vi "OAT Spectral Map (Waterfall).vi"(0 "scaled signal [EU]":waveform(dbl)={"t0"=timestamp(0 s since 1904-01-01), "dt"=0.0, "Y"=[]}, 1 "dB on? (F)":bool, 2 "reset? (F)":bool, 3 "plot type":T10(ring), 5 "speed profile":T9 {"speed [RPM]" format="%.2f"; "time [s]" format="%.2f"}, 7 "pulse/revolution (1)":i32=1, 9 "time/speed segment [s or RPM]":cluster{"start":dbl, "end":dbl, "step size":dbl} {"step size" format="%.2f"; "end" min=0.0 format="%.2f"; "start" min=0.0 format="%.2f"}, 11 "error in (no error)":errorcluster, 12 "max order (auto)":dbl, 13 "windows info":cluster{"window type":u32, "window length":i32}={"window type"=62, "window length"=2048} {"window length" min=2; "window type" items=["None"=0, "Hanning"=1, "Hamming"=2, "Blackman-Harris"=3, "Exact Blackman"=4, "Blackman"=5, "Flat Top"=6, "4 Term B-Harris"=7, "7 Term B-Harris"=8, "Low Sidelobe"=9, "Gaussian"=62]}) -> (4 "waterfall graph":T1, 6 "waterfall unit labels":T8, 8 "spectrum info":T2={"channel name"="", "description"="", "x-axis units"=0, "spectral info"={"spectrum type"=enum."Power [Magnitude^2]", "linear/dB"=enum."linear", "window"=0, "window size"=0, "FFT size"=0}, "engineering units"=0, "custom label"="", "dB reference [EU]"=0.0, "peak units"=enum."rms", "weighting filter"=0, "spectral density?"=FALSE, "unit label"="", "spectrum skewed?"=FALSE, "complimentary spectrum units"=enum."none"} {"x-axis units" items=["Time (s)"=0, "Frequency-CB (Hz)"=1, "Frequency-CPB (Hz)"=1248, "Frequency-Arbitrary (Hz)"=2357, "Quefrency (s)"=2, "Revolutions (rev)"=3, "Order"=4, "Speed (RPM)"=11, "Speed (rad/s)"=21, "Index"=65535]; "weighting filter" items=["Linear", "A-weighting", "B-weighting", "C-weighting", "ITU-R 468-4", "Dolby", "CCITT", "C-message", "Wb", "Wc", "Wd", "We", "Wf", "Wh", "Wj", "Wk", "Wm", "AES17 20 kHz lowpass", "AES17 40 kHz lowpass", "AES17 20 kHz highpass", "AES17 40 kHz highpass"]; "dB reference [EU]" format="%.2f"; "engineering units" items=["custom..."=0, "V"=1, "A"=21, "C"=30, "pC"=31, "s"=32, "-"=29, "Pa"=2, "N"=20, "g"=3, "m/s^2"=4, "m/s"=5, "m"=6, "mm/s"=12, "mm"=13, "micron/s"=14, "micron"=15, "in/s^2"=7, "in/s"=8, "in"=9, "mil/s"=10, "mil"=11, "rad/s^2"=16, "rad/s"=17, "rad"=18, "deg/s^2"=26, "deg/s"=27, "deg"=28, "RPM"=22, "cycle/s^2"=23, "Hz"=24, "cycle"=25, "strain"=19]; "spectral info"."window" items=["None "=0, "Hanning"=1, "Hamming"=2, "Blackman-Harris"=3, "Exact Blackman"=4, "Blackman"=5, "Flat Top"=6, "4 Term B-Harris "=7, "7 Term B-Harris"=8, "Low Sidelobe"=9, "Force - Exponential"=10, "Gaussian"=62]}, 10 "end reached?":bool, 15 "error out":errorcluster)   [LabVIEW 2017, in "SoundVib_OrderTracking.lvlib"]
doc: "Computes a spectral map of the <B>scaled signal [EU]</B> as a function of time or rotational speed. This VI can return the spectral map as a 2D numeric array, a colormap, or a waterfall graph. Wire data to the <B>scaled signal [EU]</B> input to determine the polymorphic instance to use or manually select the instance."
uses:
  <vilib>/addons/Sound and Vibration/Order Analysis/Resample Order Tracking/SoundVib_OrderTracking.lvlib
  <vilib>/addons/Sound and Vibration/Order Analysis/Tach Process/SubVIs/speed profile.ctl
  <vilib>/addons/_NISVFA/_Shared subVIs/Controls/svc_Spectrum Info.ctl
  <vilib>/addons/_NISVFA/_Shared subVIs/Controls/svc_X-Axis Units.ctl
  <vilib>/addons/_NISVFA/_Shared subVIs/Controls/svc_Spectrum Type.ctl
  <vilib>/addons/_NISVFA/_Shared subVIs/Controls/svc_Engineering Units Text Ring.ctl
  <vilib>/addons/_NISVFA/_Shared subVIs/Controls/svc_Weighting Filter Text Ring.ctl
  <vilib>/addons/_NISVFA/_Shared subVIs/Controls/svc_Complimentary Spectrum Units.ctl
  <vilib>/addons/_NISVFA/_Shared subVIs/Common/svc_Check for Waveform Parameter Continuity (no state).vi
  <vilib>/addons/Sound and Vibration/Order Analysis/Resample Order Tracking/OAT Convert to Even Angle Signal (1 Channel).vi
  <vilib>/Waveform/WDTOps.llb/WDT Waveform Duration DBL.vi
  <vilib>/addons/_NISVFA/_Shared subVIs/Common/svc_Engineering Units to Unit Label.vi
  <vilib>/addons/_NISVFA/_Shared subVIs/Common/svc_Unit Label to Engineering Units.vi
  <vilib>/addons/Sound and Vibration/Order Analysis/Resample Order Tracking/SoundVib_Resampling.lvlib
  <vilib>/addons/Sound and Vibration/Order Analysis/Tach Process/SoundVib_TachProcess.lvlib
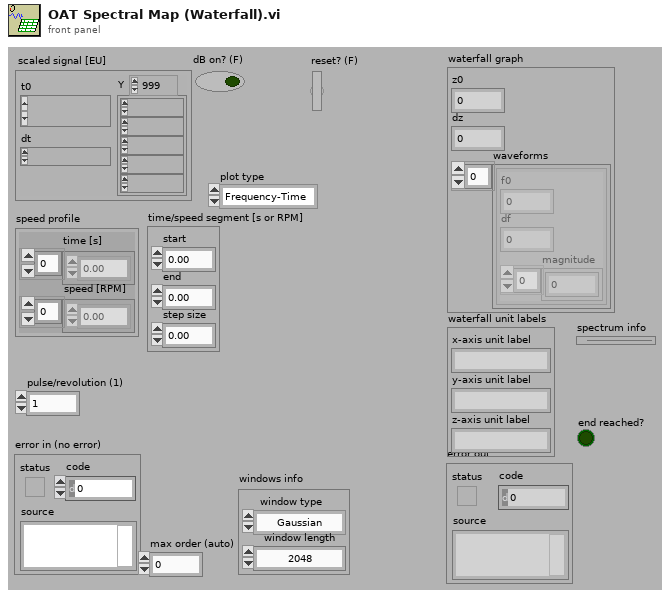
[diagram p1: front panel]
types:
  T1 = cluster{"z0":dbl, "dz":dbl, "waveforms":cluster{"f0":dbl, "df":dbl, "magnitude":dbl[]}[]}
  T2 = typedef "svc_Spectrum Info.ctl" = cluster{"channel name":string, "description":string, "x-axis units":T3, "spectral info":cluster{"spectrum type":T4, "linear/dB":enum16{"linear", "dB"}, "window":u16, "window size":i32, "FFT size":i32}, "engineering units":T5, "custom label":string, "dB reference [EU]":dbl, "peak units":enum16{"rms", "peak", "peak-peak"}, "weighting filter":T6, "spectral density?":bool, "unit label":string, "spectrum skewed?":bool, "complimentary spectrum units":T7}
  T3 = typedef "svc_X-Axis Units.ctl" = u16
  T4 = typedef "svc_Spectrum Type.ctl" = enum16{"FFT Spectrum [complex]", "Amplitude [Magnitude]", "Power [Magnitude^2]", "Cross Spectrum [complex]", "Frequency Response [Complex]"}
  T5 = typedef "svc_Engineering Units Text Ring.ctl" = u16
  T6 = typedef "svc_Weighting Filter Text Ring.ctl" = u16
  T7 = typedef "svc_Complimentary Spectrum Units.ctl" = enum16{"none", "radians", "degrees", "cycles", "imaginary"}
  T8 = cluster{"x-axis unit label":string, "y-axis unit label":string, "z-axis unit label":string}
  T9 = typedef "SoundVib_TachProcess.lvlib/speed profile.ctl" = cluster{"time [s]":dbl[], "speed [RPM]":dbl[]}
  T10 = enum16{"Frequency-Time", "Time-Frequency", "Order-Time", "Time-Order", "Frequency-RPM", "RPM-Frequency", "Order-RPM", "RPM-Order"}
  T11 = cluster{"dt":bool, "t0 continuity":bool, "array length":bool, "channel info":bool, "name":bool}
  T12 = cluster{"start (s)":dbl, "end (s)":dbl, "step (s)":dbl}
  T13 = typedef "svc_Channel Info.ctl" = cluster{"sensor sensitivity":dbl, "engineering units":T5, "dB reference":dbl, "custom label":string, "weighting filter":T6, "pregain":dbl}
  T14 = cluster{"X scale":cluster{"offset":dbl, "multiplier":dbl}, "Y scale":cluster{"offset":dbl, "multiplier":dbl}}
  T15 = cluster{"X axis unit label":string, "Y axis unit label":string, "Z axis unit label":string}
  T16 = cluster{"z0":dbl, "dz":dbl, "Waveforms":cluster{"f0":dbl, "df":dbl, "magnitude":dbl[]}[]}
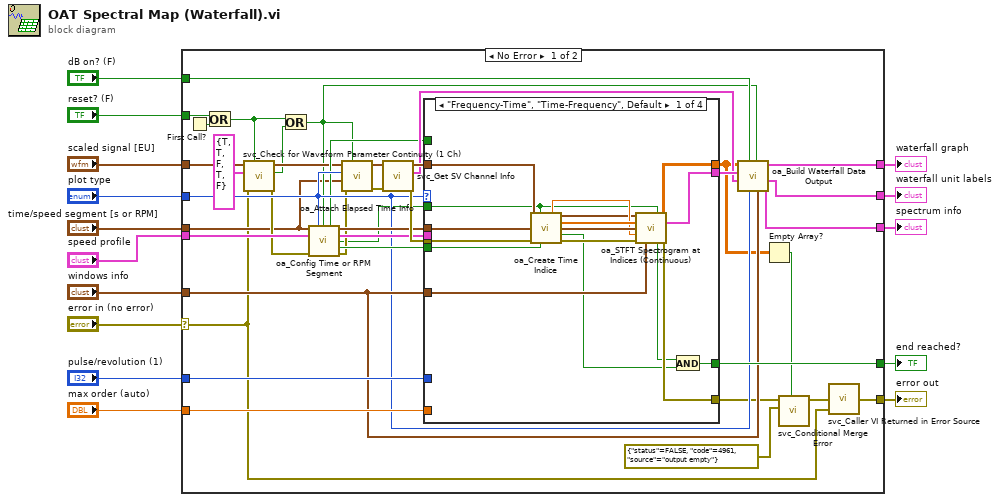
[diagram p0: block diagram]
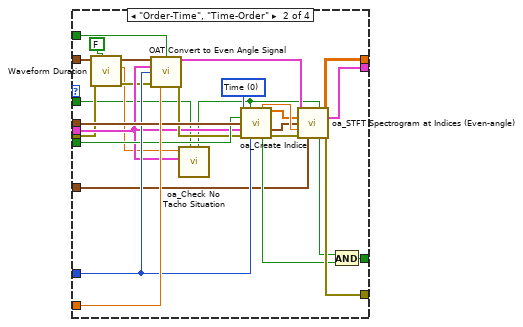
[diagram p2: hidden frame]
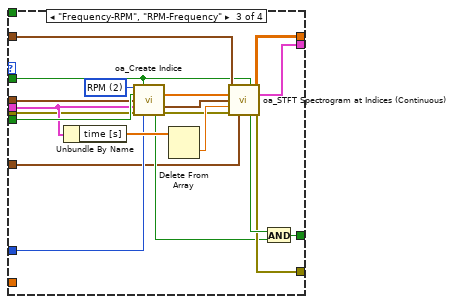
[diagram p3: hidden frame]
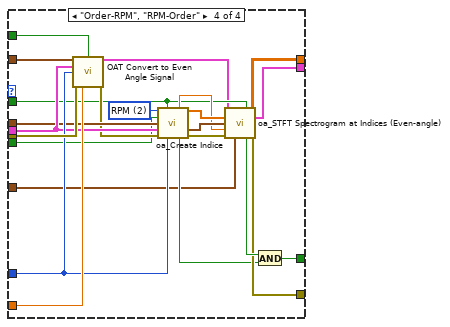
[diagram p4: hidden frame]
diagram:
  n1 = case shown="No Error" "error in (no error)" {
    selector: "error in (no error)" -> [w18 w143]
    tunnel: [w16 w143] -> w15
    tunnel: "time/speed segment [s or RPM]" -> [w23 _]
    tunnel: "scaled signal [EU]" -> [w30 _]
    tunnel: [w54 _] -> w12
    tunnel: "windows info" -> [w37 _]
    tunnel: "speed profile" -> [w41 _]
    tunnel: "pulse/revolution (1)" -> [w53 _]
    tunnel: "max order (auto)" -> [w52 _]
    tunnel: "reset? (F)" -> [w51 _]
    tunnel: "dB on? (F)" -> [w50 _]
    tunnel: [w49 _] -> w1
    tunnel: "plot type" -> [w35 _]
    tunnel: [w47 _] -> w3
    tunnel: [w46 _] -> w2
    frame No Error {
      n2 = First Call?() -> (First Call?: T/F=w48:bool)
      n3 = Or(x=w51, y=w48) -> (x .or. y?=w26:bool)
      n4 = call <vilib>:"svc_Check for Waveform Parameter Continuity (1 Ch).vi"("restart averaging (F)"=w26, "error in (no error)"=w18, "checks for channel parameter change"=T11 {"dt"=TRUE, "t0 continuity"=TRUE, "array length"=FALSE, "channel info"=TRUE, "name"=FALSE}, "scaled signal [EU]"=w30) -> ("error out"=w29:errorcluster, "waveform parameter changed"=w25:bool, "dup scaled signal [EU]"=w28:waveform(dbl))  [unwired: 2 in, 3 out]
      n5 = Or(x=w26, y=w25) -> (x .or. y?=w24:bool)
      n6 = call <vilib>:"oa_Config Time or RPM Segment.vi"("time segment"=w23, "plot type"=w35, "reset in"=w24, "speed profile"=w41, "error in (no error)"=w29) -> ("reset resampling"=w31:bool, "time segment out"=w40:T12, "speed profile out"=w39:T9, "reset out"=w32:bool, "step found?"=w38:bool, "error out"=w34:errorcluster)  [unwired: 5 in]
      n7 = call <vilib>:"oa_Attach Elapsed Time Info.vi"("reset? (F)"=w24, "error in (no error)"=w34, "time/speed segment [s or rpm]"=w23, "plot type"=w35, "scaled signal [EU]"=w28) -> ("error out"=w33:errorcluster, "scaled signal [EU] out"=w36:waveform(dbl))  [unwired: 5 in]
      n8 = call <vilib>:"svc_Get SV Channel Info.vi"("error in (no error)"=w33, "scaled signal [EU]"=w36) -> ("error out"=w44:errorcluster, "channel info"=w42:T13, "dup scaled signal [EU]"=w45:waveform(dbl))  [unwired: 4 in, 3 out]
      n9 = case shown="\"Frequency-Time\", \"Time-Frequency\", Default" w35 {
        tunnel: w45 -> [w57 w95 w106 w135]
        tunnel: w40 -> [w63 w88 w112 w130]
        tunnel: [w71 w97 w118 w142] -> w20
        tunnel: [w70 w96 w117 w141] -> w43
        tunnel: [w69 w98 w115 w138] -> w21
        tunnel: [w67 w93 w116 w139] -> w54
        tunnel: w44 -> [w56 w77 w102 w137]
        tunnel: w39 -> [_ w79 w111 w131]
        tunnel: w53 -> [_ w87 w105 w132]
        tunnel: w52 -> [_ w99 _ w136]
        tunnel: w38 -> [w64 w86 w114 w124]
        tunnel: w37 -> [w66 w83 w103 w123]
        tunnel: w32 -> [w55 w73 w100 w122]
        tunnel: w31 -> [_ w81 _ w121]
        frame "Frequency-Time", "Time-Frequency", Default {
          n10 = call <vilib>:"oa_Create Time Indice.vi"("scaled signal [EU]"=w57, "reset? (True)"=w55, "steps"=w63, "error in (no error)"=w56, "step found?(F)"=w64) -> ("signal processed"=w59:dbl, "scaled signal [EU] dup"=w58:waveform(dbl), "time indices"=w62:dbl[], "scale"=w61:cluster{"offset":dbl, "multiplier":dbl}, "finished?"=w60:bool, "error out"=w65:errorcluster)  [unwired: 5 in]
          n11 = call <vilib>:"oa_STFT Spectrogram at Indices (Continuous).vi"("resampled signal"=w58, "reset? (True)"=w55, "time indices"=w62, "X scale in"=w61, "last indices"=w59, "error in (no error)"=w65, "spectral settings"=w66) -> ("spectral map"=w71:dbl[][], "scales"=w70:T14, "finished"=w68:bool, "error out"=w69:errorcluster)  [unwired: 5 in]
          n12 = And(x=w68, y=w60) -> (x .and. y?=w67:bool)
        }
        frame "Order-Time", "Time-Order" {
          w92 = u16 0 items=["Time", "Revolution", "RPM"] ("X axis selection")
          n13 = call-poly <vilib>:"Waveform Duration.vi"("open interval? (T)"=FALSE, "error in (no error)"=w77, "waveform in"=w95) -> ("error out"=w76:errorcluster, "duration"=w74:dbl, "waveform out"=w78:waveform(dbl))  [unwired: 6 in]
          n14 = call-poly <vilib>:"OAT Convert to Even Angle Signal.vi"("scaled signal [EU]"=w78, "reset? (F)"=w81, "speed profile"=w79, "pulse/revolution (1)"=w87, "error in (no error)"=w76, "max order (auto)"=w99) -> ("even-angle signal"=w80:cluster{"r0":dbl, "dr":dbl, "Y":dbl[]}, "error out"=w85:errorcluster)  [unwired: 5 in, 3 out]
          n15 = call <vilib>:"oa_Check No Tacho Situation.vi"("reset in"=w73, "speed profile"=w79, "input duration"=w74) -> ("reset out"=w72:bool)  [unwired: 8 in]
          n16 = call <vilib>:"oa_Create Indice.vi"("X axis selection"=w92, "reset?(F)"=w72, "step found?(F)"=w86, "steps input"=w88, "speed profile"=w79, "error in (no error)"=w85, "pulse/revolution (1)"=w87) -> ("last rev"=w90:dbl, "rev indice"=w82:dbl[], "scale"=w89:cluster{"offset":dbl, "multiplier":dbl}, "reach end?"=w91:bool, "error out"=w84:errorcluster)  [unwired: 2 in, 2 out]
          n17 = call <vilib>:"oa_STFT Spectrogram at Indices (Even-angle).vi"("even-angle signal"=w80, "reset? (True)"=w72, "rev indices"=w82, "X scale in"=w89, "last indices"=w90, "error in (no error)"=w84, "spectral settings"=w83) -> ("spectral map"=w97:dbl[][], "scales"=w96:T14, "finished"=w94:bool, "error out"=w98:errorcluster)  [unwired: 5 in]
          n18 = And(x=w94, y=w91) -> (x .and. y?=w93:bool)
        }
        frame "Frequency-RPM", "RPM-Frequency" {
          w113 = u16 2 items=["Time", "Revolution", "RPM"] ("X axis selection")
          n19 = Unbundle By Name(w111) -> ("time [s]"=w108:dbl[])
          n20 = call <vilib>:"oa_Create Indice.vi"("X axis selection"=w113, "reset?(F)"=w100, "step found?(F)"=w114, "steps input"=w112, "speed profile"=w111, "error in (no error)"=w102, "pulse/revolution (1)"=w105) -> ("time indice"=w110:dbl[], "scale"=w109:cluster{"offset":dbl, "multiplier":dbl}, "reach end?"=w104:bool, "error out"=w101:errorcluster)  [unwired: 2 in, 3 out]
          n21 = Delete From Array(array=w108) -> (deleted portion=w107:dbl)  [unwired: 2 in, 1 out]
          n22 = call <vilib>:"oa_STFT Spectrogram at Indices (Continuous).vi"("resampled signal"=w106, "reset? (True)"=w100, "time indices"=w110, "X scale in"=w109, "last indices"=w107, "error in (no error)"=w101, "spectral settings"=w103) -> ("spectral map"=w118:dbl[][], "scales"=w117:T14, "finished"=w119:bool, "error out"=w115:errorcluster)  [unwired: 5 in]
          n23 = And(x=w119, y=w104) -> (x .and. y?=w116:bool)
        }
        frame "Order-RPM", "RPM-Order" {
          w134 = u16 2 items=["Time", "Revolution", "RPM"] ("X axis selection")
          n24 = call-poly <vilib>:"OAT Convert to Even Angle Signal.vi"("scaled signal [EU]"=w135, "reset? (F)"=w121, "speed profile"=w131, "pulse/revolution (1)"=w132, "error in (no error)"=w137, "max order (auto)"=w136) -> ("even-angle signal"=w120:cluster{"r0":dbl, "dr":dbl, "Y":dbl[]}, "error out"=w126:errorcluster)  [unwired: 5 in, 3 out]
          n25 = call <vilib>:"oa_Create Indice.vi"("X axis selection"=w134, "reset?(F)"=w122, "step found?(F)"=w124, "steps input"=w130, "speed profile"=w131, "error in (no error)"=w126, "pulse/revolution (1)"=w132) -> ("last rev"=w127:dbl, "rev indice"=w128:dbl[], "scale"=w129:cluster{"offset":dbl, "multiplier":dbl}, "reach end?"=w133:bool, "error out"=w125:errorcluster)  [unwired: 2 in, 2 out]
          n26 = call <vilib>:"oa_STFT Spectrogram at Indices (Even-angle).vi"("even-angle signal"=w120, "reset? (True)"=w122, "rev indices"=w128, "X scale in"=w129, "last indices"=w127, "error in (no error)"=w125, "spectral settings"=w123) -> ("spectral map"=w142:dbl[][], "scales"=w141:T14, "finished"=w140:bool, "error out"=w138:errorcluster)  [unwired: 5 in]
          n27 = And(x=w140, y=w133) -> (x .and. y?=w139:bool)
        }
      }
      n28 = call <vilib>:"oa_Build Waterfall Data Output.vi"("windows info"=w37, "reset? (F)"=w24, "plot type"=w35, "dB on"=w50, "channel info"=w42, "scales"=w43, "spectral map"=w20) -> ("spectrum info out"=w46:T2, "waterfall unit labels"=w47:T15, "Waterfall Graph"=w49:T16)  [unwired: 2 in]
      n29 = Empty Array?(array=w20) -> (empty?=w19:bool)
      n30 = call <vilib>:"svc_Conditional Merge Error.vi"("merge"=w19, "new error"=errorcluster {"status"=FALSE, "code"=4961, "source"="output empty"}, "error in (no error)"=w21) -> ("error out"=w17:errorcluster)  [unwired: 8 in]
      n31 = call <vilib>:"svc_Caller VI Returned in Error Source.vi"("warning input to caller"=w18, "error in (no error)"=w17) -> ("error out"=w16:errorcluster)  [unwired: 3 in]
    }
    frame Error {
    }
  }
  "end reached?" <- w12
  "error out" <- w15
  "waterfall unit labels" <- w3
  "spectrum info" <- w2
  "waterfall graph" <- w1
